vi "Retrieve Actual OD Values.vi"(8 "error in":errorcluster, 11 "Interactor in":refnum<class "Interactor.lvclass">) -> (0 "error out":errorcluster, 3 "Interactor out":refnum<class "Interactor.lvclass">)   [LabVIEW 2024]
uses:
  Interactor.lvclass
  Interactor.lvclass/Interactor.ctl
  EDS-File-Viewer/Electronic Datasheet/Electronic Datasheet.lvclass
  C:/Program Files/National Instruments/LabVIEW 2025/vi.lib/MGI/Panel Manager/Panel Actor/Panel Actor/Panel Actor.lvclass
  C:/Program Files/National Instruments/LabVIEW 2025/vi.lib/ActorFramework/Actor/Actor.lvclass
  D:/git/CANopen-XNET/Example/Interactor/Interactor.lvclass
panel:
  out "Values":T1(array[cluster])
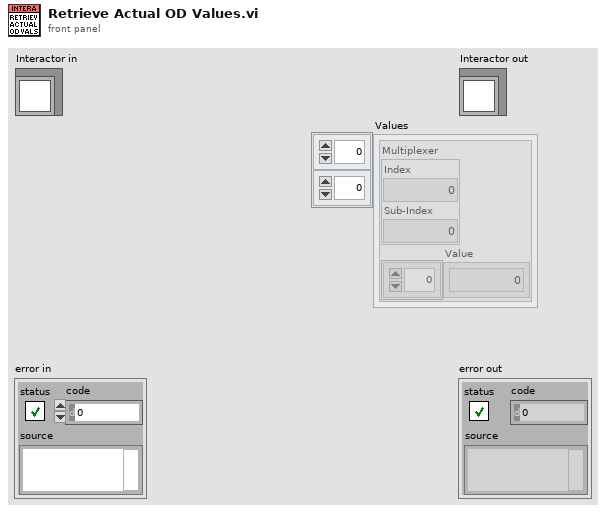
[diagram p1: front panel]
types:
  T1 = cluster{"Multiplexer":cluster{"Index":u16, "Sub-Index":u8}, "Value":u8[]}[][]
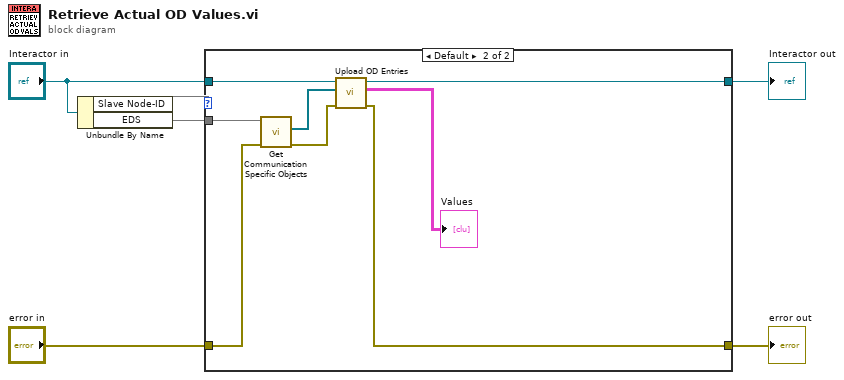
[diagram p0: block diagram]
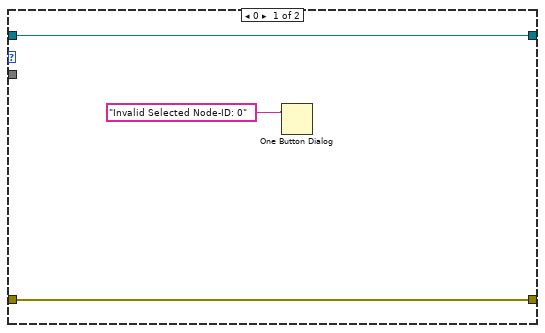
[diagram p2: hidden frame]
diagram:
  n1 = Unbundle By Name("Interactor in") -> ("Slave Node-ID"=w1, "EDS"=w6)
  n2 = case shown="Default" w1 {
    tunnel: w6 -> [_ w14]
    tunnel: "error in" -> [w9 w13]
    tunnel: "Interactor in" -> [w7 w12]
    tunnel: [w7 w11] -> w3
    tunnel: [w9 w10] -> w2
    frame 0 {
      n3 = One Button Dialog(message="Invalid Selected Node-ID: 0") -> ()  [unwired: 1 in, 1 out]
    }
    frame Default {
      n4 = call "Get Communication Specific Objects.vi"("error in"=w13, "Electronic Datasheet"=w14) -> ("error out"=w16:errorcluster, "Entries"=w17:refnum<class "OD Entry.lvclass">[])  [unwired: 7 in, 1 out]
      n5 = call-dynamic "Upload OD Entries.vi"("error in"=w16, "Entries"=w17, "Interactor in"=w12) -> ("error out"=w10:errorcluster, "Values"=→"Values":T1, "Interactor out"=w11:refnum<class "Interactor.lvclass">)  [unwired: 6 in]
    }
  }
  "error out" <- w2
  "Interactor out" <- w3
